vi "Num-StringToDecNum.vi"(0 "Sting Num In":string) -> (5 "Number Out":i32)   [LabVIEW 2013]
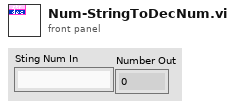
[diagram p1: front panel]
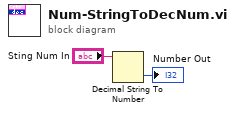
[diagram p0: block diagram]
diagram:
  n1 = Decimal String To Number(string="Sting Num In") -> (number=→"Number Out":i32)  [unwired: 2 in, 1 out]
